vi "Array Restructure.vi"() -> ()   [LabVIEW 2016]
panel:
  out "Parsed CMD Array":u16[](array[numeric]) format="%04x"
  out "Parsed Data Array":u16[](array[numeric]) format="%04x"
  in  "Subset Size":i32=8
  in  "Original Array":u16[](array[numeric])=[4660, 22136, 43981, 4369, 17185, 34661, 43981, 8738, 8500, 25976, 56506, 13107, 30296, 12820, 56506, 17476] format="%04x"
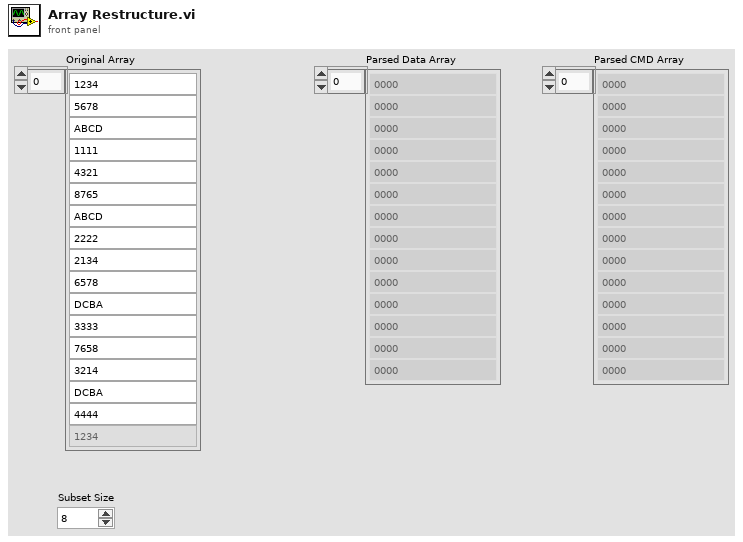
[diagram p1: front panel]
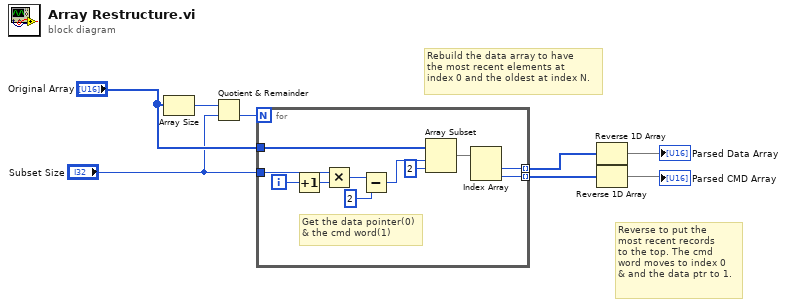
[diagram p0: block diagram]
diagram:
  # "Reverse to put the\nmost recent records\nto the top. The cmd\nword moves to index 0\n& and the data ptr to 1."
  # "Rebuild the data array to have\nthe most recent elements at\nindex 0 and the oldest at index N."
  n1 = Array Size(array="Original Array") -> (size(s)=w8:i32)
  n2 = Quotient & Remainder(x=w8, y="Subset Size") -> (floor(x/y)=w6:i32)  [unwired: 1 out]
  n3 = for {
    N: w6 -> [_]
    tunnel: "Original Array" -> [w19]
    tunnel: "Subset Size" -> [w18]
    tunnel: [w10] -> w3 mode=indexing
    tunnel: [w9] -> w2 mode=indexing
    i -> [w16]
    # "Get the data pointer(0)\n& the cmd word(1)"
    n4 = Increment(x=w16) -> (x+1=w15:i32)
    n5 = Multiply(x=w18, y=w15) -> (x*y=w14:i32)
    n6 = Subtract(x=w14, y=2 ("length")) -> (x-y=w12:i32)
    n7 = Array Subset(array=w19, index=w12, length=2) -> (w11:u16[])
    n8 = Index Array(array=w11) -> (element #1=w10:u16, element #2=w9:u16)  [unwired: 2 in]
  }
  n9 = Reverse 1D Array(array=w3) -> (reversed array=→"Parsed Data Array":u16[])
  n10 = Reverse 1D Array(array=w2) -> (reversed array=→"Parsed CMD Array":u16[])
